vi "test_Delete Instrument Addon.vi"(8 "error in (no error)":errorcluster, 11 "TestCase in":refnum<class "Instrument Addon Scripting API Custom Device Unit Tests.lvclass">) -> (0 "error out":errorcluster, 3 "TestCase out":refnum<class "Instrument Addon Scripting API Custom Device Unit Tests.lvclass">)   [LabVIEW 2018, in "Instrument Addon Scripting API Custom Device Unit Tests.lvclass"]
uses:
  Instrument Addon Scripting API Custom Device Unit Tests.lvclass
  NationalInstruments.VeriStand.SystemDefinitionAPI
  Instrument Addon Scripting API Custom Device Unit Tests.lvclass/Instrument Addon Scripting API Custom Device Unit Tests.ctl
  Addon/Addon Shared/SubVIs/Constants.vi
  <vilib>/addons/_JKI Toolkits/VI Tester/TestCase.llb/TestCase.lvclass
  Instrument Addon Scripting API Test Assets/Instrument Addon Scripting API Test Assets.lvclass
  APIs/Scripting API/Instrument Addon Scripting API.lvlib
  Addon/Addon Shared/Instrument Addon Shared.lvlib
  C:/Program Files (x86)/National Instruments/LabVIEW 2018/vi.lib/addons/_JKI Toolkits/VI Tester/TestCase.llb/TestCase.lvclass
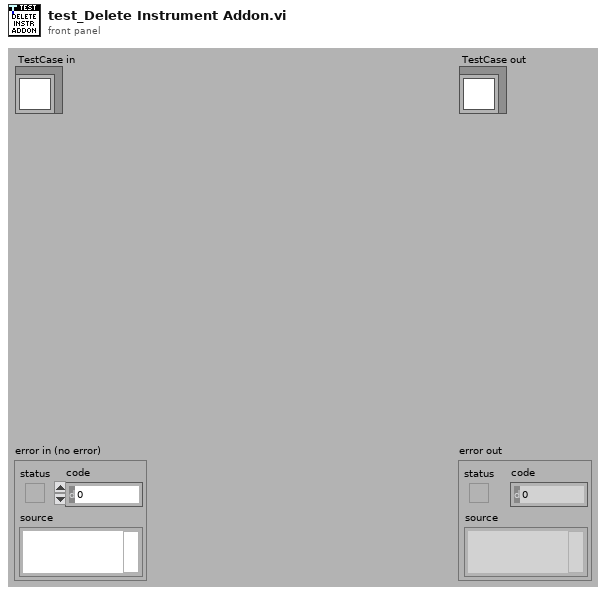
[diagram p1: front panel]
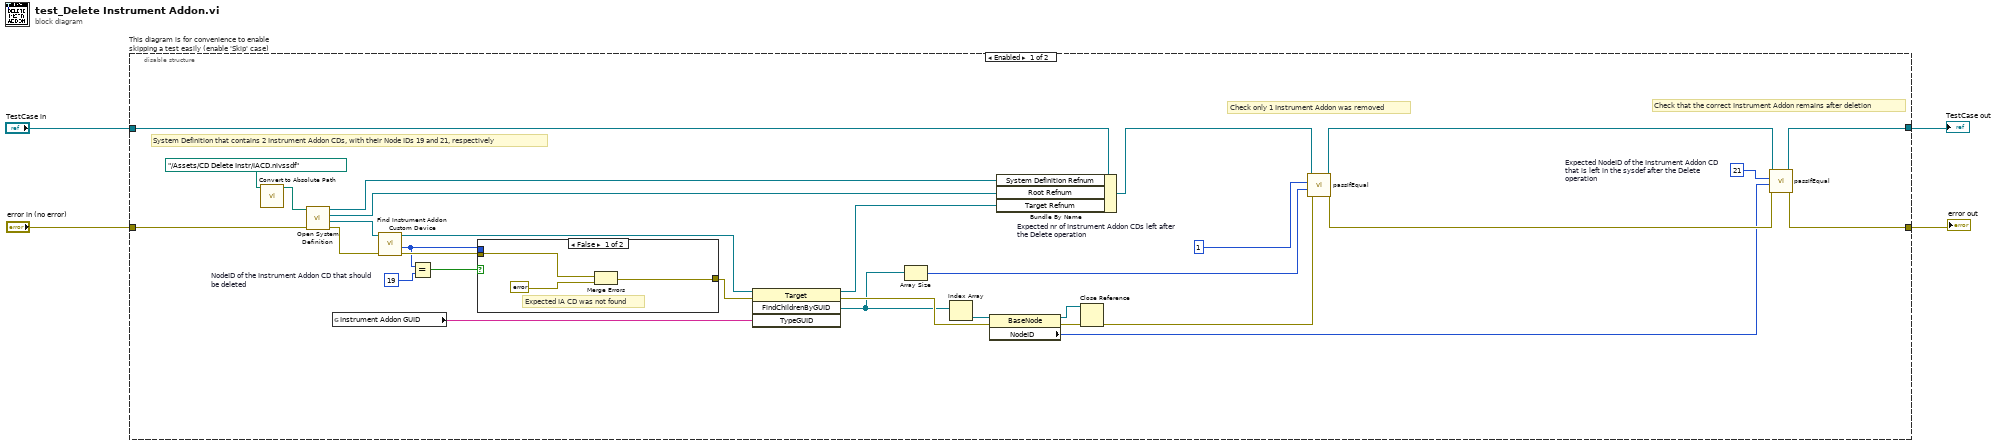
[diagram p0: block diagram]
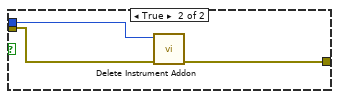
[diagram p2: hidden frame]
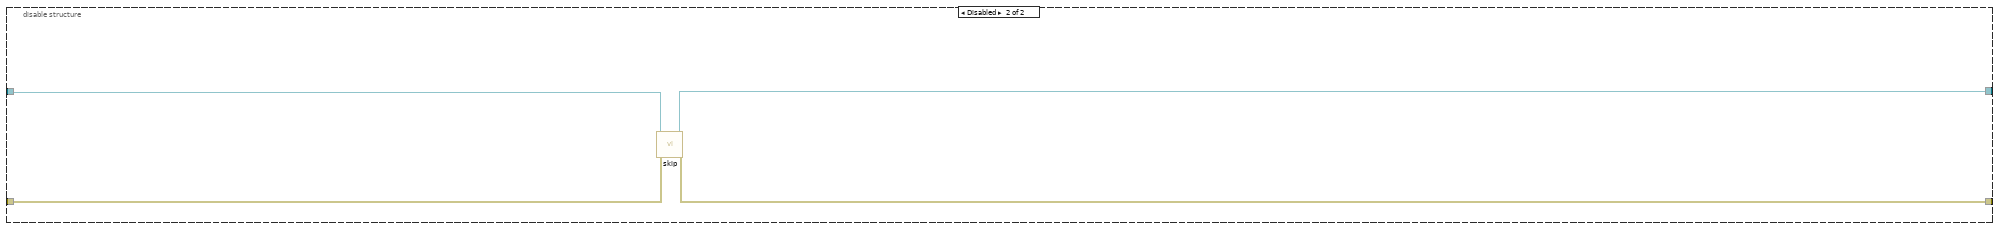
[diagram p3: hidden frame]
diagram:
  n1 = disable-structure "This diagram is for convenience to enable skipping a test easily (enable 'Skip' case)" shown="Enabled" {
    disable-tunnel: "TestCase in" -> [w12 w43]
    disable-tunnel: [w32 w42] -> w1
    disable-tunnel: [w33 w45] -> w3
    disable-tunnel: "error in (no error)" -> [w35 w44]
    frame Enabled {
      w15 = 1  # Expected nr of Instrument Addon CDs left after the Delete operation
      w19 = u64 21  # Expected NodeID of the Instrument Addon CD that is left in the sysdef after the Delete operation
      w25 = u64 19  # NodeID of the Instrument Addon CD that should be deleted
      # "Check only 1 Instrument Addon was removed"
      # "System Definition that contains 2 Instrument Addon CDs, with their Node IDs 19 and 21, respectively"
      # "Check that the correct Instrument Addon remains after deletion"
      n2 = call "Convert to Absolute Path.vi"("System Definition File"=path "../Assets/CD Delete Instr/IACD.nivssdf" ("SDF file")) -> ("Absolute Path"=w34:path)  [unwired: 10 in]
      n3 = call "Open System Definition.vi"("error in (no error)"=w35, "System Definition File"=w34) -> ("error out"=w31:errorcluster, "Target Refnum"=w23:refnum<k24>, "Root Refnum"=w10:refnum<k24>, "System Definition Refnum"=w11:refnum<k24>)  [unwired: 6 in]
      n4 = global read "Constants.vi" "Instrument Addon GUID"() -> (w22:string)
      n5 = call "Find Instrument Addon Custom Device.vi"("error in"=w31, "target in"=w23) -> ("error out"=w30:errorcluster, "NodeID"=w26:u64, "target out"=w27:refnum<k24>)  [unwired: 7 in]
      n6 = Equal?(x=w26, y=w25) -> (x = y?=w24:bool)
      n7 = case shown="False" w24 {
        tunnel: w30 -> [w38 w41]
        tunnel: [w36 w40] -> w29
        tunnel: w26 -> [_ w39]
        frame False {
          # "Expected IA CD was not found"
          n8 = Merge Errors(w38, errorcluster {"status"=TRUE, "code"=0, "source"="Sysdef does not contain a Instrument Addon Custom Device"} ("error out")) -> (w36:errorcluster)
        }
        frame True {
          n9 = call "Delete Instrument Addon.vi"("error in (no error)"=w41, "Instrument Addon Refnum"=w39) -> ("error out"=w40:errorcluster)  [unwired: 9 in]
        }
      }
      n10 = invoke class="Target" method="FindChildrenByGUID"(reference=w27, error in=w29, "TypeGUID"=w22) -> (reference out=w9:refnum<k24>, error out=w20:errorcluster, "FindChildrenByGUID"=w18:refnum<k24>[])  [unwired: 1 in, 1 out]
      n11 = Array Size(array=w18) -> (size(s)=w16:i32)
      n12 = Index Array(array=w18) -> (element=w21:refnum<k24>)  [unwired: 1 in]
      n13 = property class="BaseNode"(reference=w21, error in=w20) -> (reference out=w5:refnum<k24>, error out=w7:errorcluster, "NodeID"=w13:u64)
      n14 = Bundle By Name(cluster=w12, "System Definition Refnum"=w11, "Root Refnum"=w10, "Target Refnum"=w9) -> (w8:refnum<class "Instrument Addon Scripting API Custom Device Unit Tests.lvclass">)
      n15 = Close Reference(reference=w5, error in (no error)=w7) -> (error out=w6:errorcluster)
      n16 = call-dynamic "passIfEqual.vi"("error in (no error)"=w6, "y"=w16, "x"=w15, "TestCase in"=w8) -> ("error out"=w17:errorcluster, "TestCase out"=w14:refnum<class "Instrument Addon Scripting API Custom Device Unit Tests.lvclass">)  [unwired: 6 in]
      n17 = call-dynamic "passIfEqual.vi"("error in (no error)"=w17, "y"=w13, "x"=w19, "TestCase in"=w14) -> ("error out"=w33:errorcluster, "TestCase out"=w32:refnum<class "Instrument Addon Scripting API Custom Device Unit Tests.lvclass">)  [unwired: 6 in]
    }
    frame Disabled {
      # "skip test result while test is under development"
      n18 = call <vilib>:"skip.vi"("error in (no error)"=w44, "TestCase in"=w43) -> ("error out"=w45:errorcluster, "TestCase out"=w42:refnum<class "Instrument Addon Scripting API Custom Device Unit Tests.lvclass">)  [unwired: 8 in]
    }
  }
  "error out" <- w3
  "TestCase out" <- w1
